vi "高速数据通信 指令批处理.vi"() -> ()   [LabVIEW 2018]
doc: "This example mainly indicates how to acquire profiles from controllers by using <B>Read Profiles (for High-Speed Communication)</B> VI via high-speed communication."
uses:
  Public/Clusters/Ethernet Config.ctl
  Public/Clusters/High-Speed Comm Start Req.ctl
  Public/Constants/High-Speed Comm Start Pos.ctl
  Public/Constants/High-Speed Receive Ratio.ctl
  Public/Clusters/Profile Info.ctl
  KEYENCE LJ-X8000A.lvlib
panel:
  in  "Program No":u8
  in  "btnChangeProgram":bool
  in  "stop measure":bool
  in  "start measure":bool
  out "Luminance Image":u16[][](graph)
  out "error out":errorcluster
  out "Comm":bool
  out "Monitoring":bool
  out "Timeout Cnt":u32
  out "Height Image":dbl[][](graph)
  out "Read Cnt":u32
  out "Notify":u32
  out "Buf Usage Rate":u32
  out "Profile Info":T1
  in  "Start Req":T2={"High-Speed Comm Start Pos"=2, "Read Profile Cnt"=11, "High-Speed Receive Ratio"=16} {"High-Speed Receive Ratio" items=["LOWEST"=0, "LOW"=16, "MIDDLE"=17, "HIGH"=18, "HIGHEST"=32]; "High-Speed Comm Start Pos" items=["SEND COMPLETE POS", "OLDEST", "NEXT"]}
  in  "Port No":u16=24692
  in  "Stop Monitoring":bool
  in  "Start Monitoring":bool
  in  "Stop High Speed Comm":bool
  in  "Start High Speed Comm":bool
  in  "Stop VI":bool
  in  "Ethernet Config":T5={"IP Address"=[192, 168, 0, 1], "Port No"=24691}
  # "High Speed Data Communication Start/Stop"
  # "Read Profiles Start/Stop"
  # "Communication Configuration"
  # "Output from Read Profiles VI"
  # "Communication Configuration\nfor High Speed Communication"
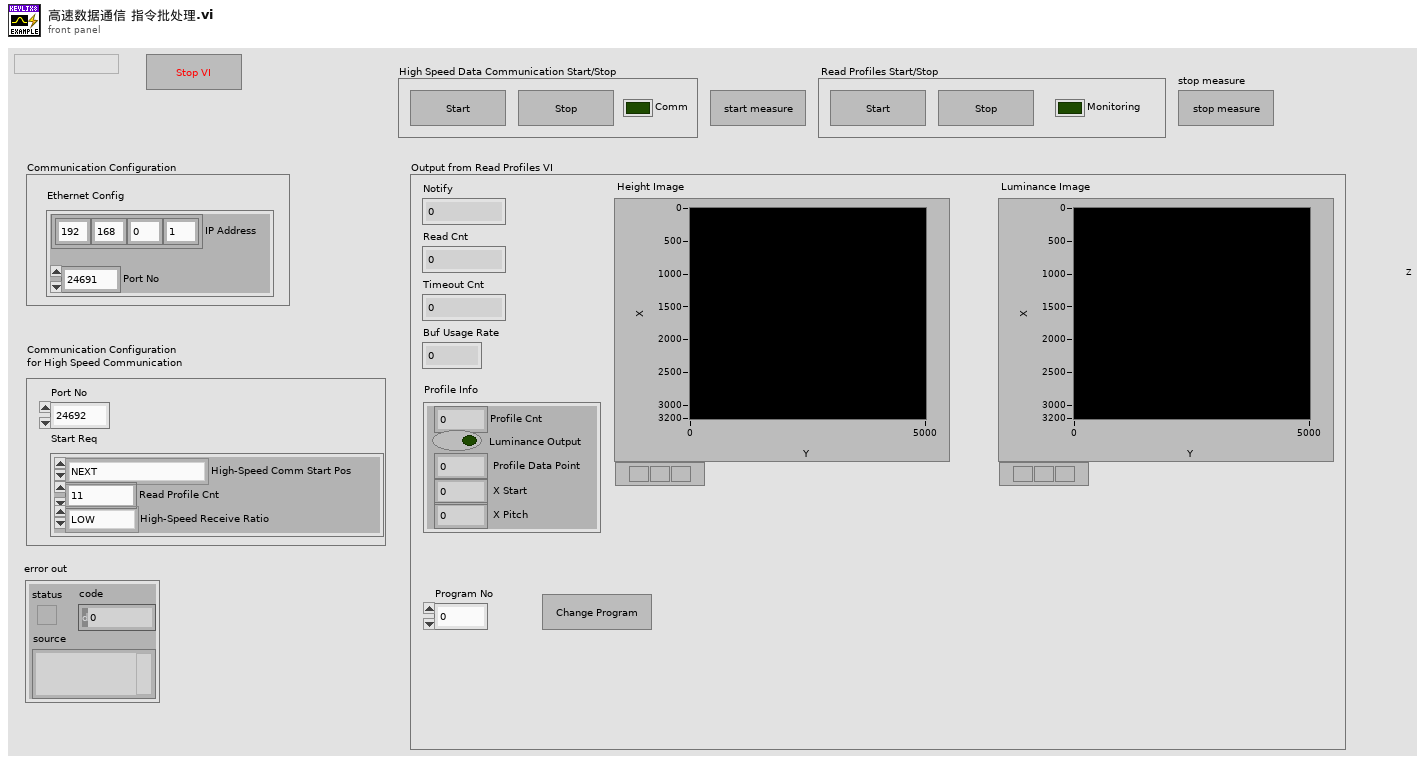
[diagram p1: front panel]
types:
  T1 = typedef "KEYENCE LJ-X8000A.lvlib/Profile Info.ctl" = cluster{"Profile Cnt":u8, "Luminance Output":bool, " Profile Data Point":u16, " X Start":i32, " X Pitch":i32}
  T2 = typedef "KEYENCE LJ-X8000A.lvlib/High-Speed Comm Start Req.ctl" = cluster{"High-Speed Comm Start Pos":T3, "Read Profile Cnt":u32, "High-Speed Receive Ratio":T4}
  T3 = typedef "KEYENCE LJ-X8000A.lvlib/High-Speed Comm Start Pos.ctl" = u8
  T4 = typedef "KEYENCE LJ-X8000A.lvlib/High-Speed Receive Ratio.ctl" = u8
  T5 = typedef "KEYENCE LJ-X8000A.lvlib/Ethernet Config.ctl" = cluster{"IP Address":u8[], "Port No":u16}
  T6 = enum8{"Enabled", "Disabled", "Disabled and Grayed Out"}
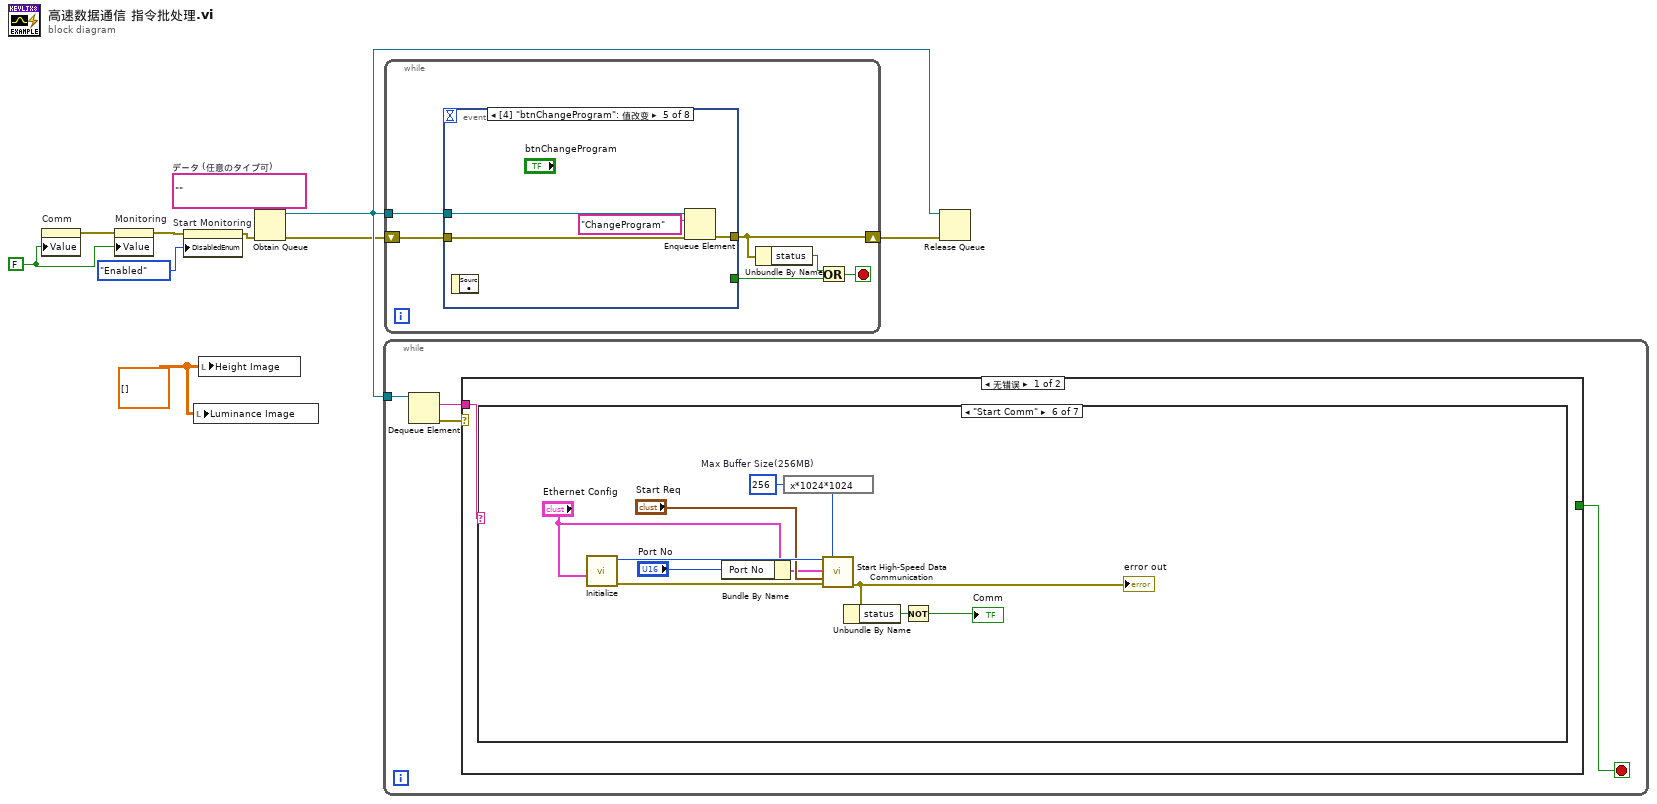
[diagram p0: block diagram]
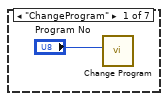
[diagram p2: hidden frame]
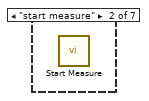
[diagram p3: hidden frame]
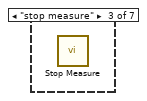
[diagram p4: hidden frame]
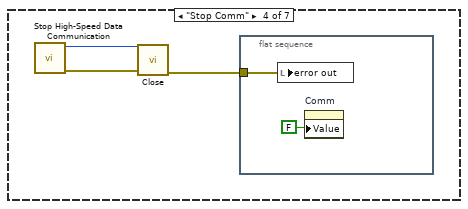
[diagram p5: hidden frame]
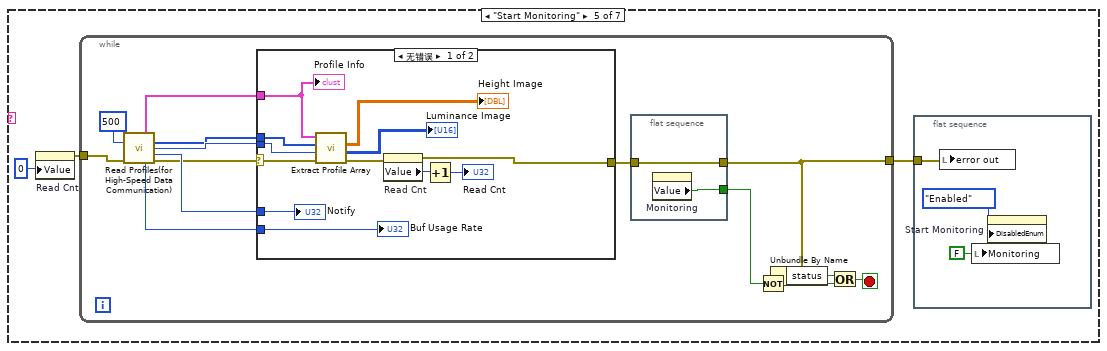
[diagram p6: hidden frame]
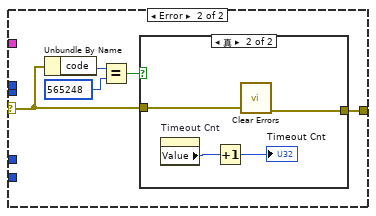
[diagram p7: hidden frame]
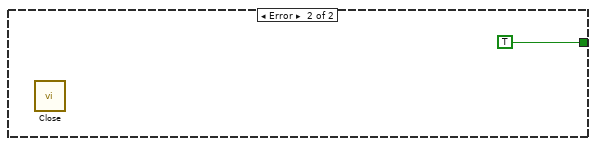
[diagram p10: hidden frame]
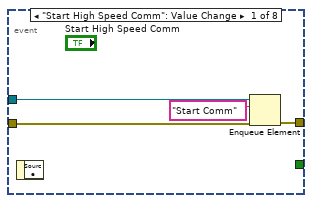
[diagram p11: hidden frame]
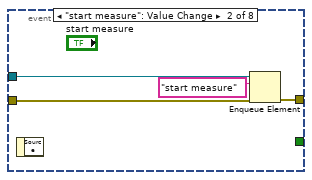
[diagram p12: hidden frame]
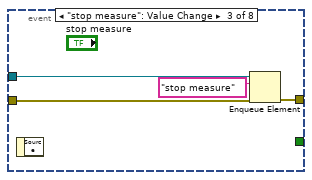
[diagram p13: hidden frame]
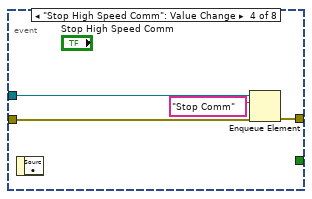
[diagram p14: hidden frame]
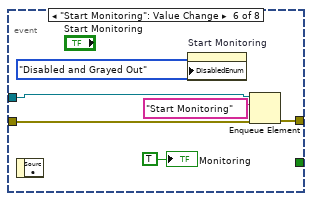
[diagram p15: hidden frame]
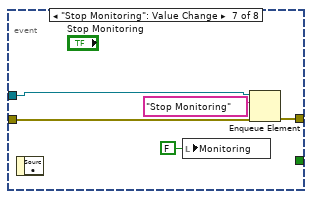
[diagram p16: hidden frame]
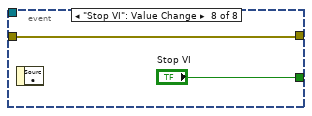
[diagram p17: hidden frame]
diagram:
  w1 = dbl[][] []
  w6 = FALSE ("Monitoring")
  w8 = ""  # データ (任意のタイプ可)
  n1 = property on="Comm" class="Bool (严格)"("Value"=w6) -> (error out=w7:errorcluster)  [unwired: 2 in, 1 out]
  n2 = property on="Monitoring" class="Bool (严格)"(error in=w7, "Value"=w6) -> (error out=w5:errorcluster)  [unwired: 1 in, 1 out]
  n3 = property on="Start Monitoring" class="Bool"(error in=w5, "DisabledEnum"=T6."Enabled" ("–³Œø")) -> (error out=w3:errorcluster)  [unwired: 1 in, 1 out]
  n4 = local write "Luminance Image"(w1) -> ()
  n5 = local write "Height Image"(w1) -> ()
  n6 = Obtain Queue(element data type=w8, error in (no error)=w3) -> (queue out=w9:refnum<queue>, error out=w4:errorcluster)  [unwired: 3 in, 1 out]
  n7 = while {
    tunnel: w9 -> [w14]
    stop <- w11 stop-if-true
    n8 = Dequeue Element(queue=w14) -> (element=w12:string, error out=w13:errorcluster)  [unwired: 2 in, 2 out]
    n9 = case shown="无错误" w13 {
      tunnel: w12 -> [w15 _]
      tunnel: [_ TRUE] -> w11
      frame No Error {
        n10 = case shown="\"Start Comm\"" w15 {
          frame "ChangeProgram" {
            n11 = call "Change Program.vi"("Program No"="Program No") -> ()  [unwired: 9 in, 2 out]
          }
          frame "start measure" {
            n12 = call "Start Measure.vi"() -> ()  [unwired: 10 in, 2 out]
          }
          frame "stop measure" {
            n13 = call "Stop Measure.vi"() -> ()  [unwired: 10 in, 2 out]
          }
          frame "Stop Comm" {
            n14 = call "Stop High-Speed Data Communication.vi"() -> ("error out"=w19:errorcluster, "Device ID out"=w18:i32)  [unwired: 10 in]
            n15 = call "Close.vi"("error in (no error)"=w19, "Device ID (0)"=w18) -> ("error out"=w17:errorcluster)  [unwired: 8 in, 1 out]
            n16 = flat-sequence {
              tunnel: w17 -> [w21]
              frame #0 {
                n17 = local write "error out"(w21) -> ()
                n18 = property on="Comm" class="Bool (严格)"("Value"=FALSE ("Comm")) -> ()  [unwired: 2 in, 2 out]
              }
            }
          }
          frame "Start Monitoring" {
            n19 = property on="Read Cnt" class="DigNum (严格)"("Value"=u32 0 ("Read Cnt")) -> (error out=w23:errorcluster)  [unwired: 2 in, 1 out]
            n20 = while {
              tunnel: w23 -> [w36]
              tunnel: [w31] -> w24
              stop <- w33 stop-if-true
              n21 = call "Read Profiles(for High-Speed Data Communication).vi"("Timeout"=u32 500, "error in (no error)"=w36) -> ("Profile Info"=w40:T1, "Profile Data"=w34:u32[], "Rsp Profile Cnt"=w37:u32, "Notify"=w38:u32, "Buf Usage Rate"=w41:u32, "error out"=w29:errorcluster)  [unwired: 7 in, 1 out]
              n22 = case shown="无错误" w29 {
                selector: w29 -> [w50 w60]
                tunnel: w41 -> [w55 _]
                tunnel: w40 -> [w49 _]
                tunnel: w38 -> [w54 _]
                tunnel: w37 -> [w47 _]
                tunnel: [w51 w59] -> w32
                tunnel: w34 -> [w48 _]
                frame No Error {
                  n23 = call "Extract Profile Array.vi"("error in (no error)"=w50, "Profile Cnt"=w47, "Profile Data"=w48, "Profile Info"=w49) -> ("error out"=w46:errorcluster, "Luminance Profile Array"=→"Luminance Image":u16[][], "Height Profile Array"=→"Height Image":dbl[][])  [unwired: 4 in, 1 out]
                  n24 = property on="Read Cnt" class="DigNum (严格)"(error in=w46) -> (error out=w51:errorcluster, "Value"=w53:u32)  [unwired: 1 in, 1 out]
                  n25 = Increment(x=w53) -> (x+1=→"Read Cnt":u32)
                  "Buf Usage Rate" <- w55
                  "Profile Info" <- w49
                  "Notify" <- w54
                }
                frame Error {
                  n26 = Unbundle By Name(w60) -> ("code"=w58:i32)
                  n27 = Equal?(x=w58, y=565248) -> (x = y?=w56:bool)
                  n28 = case shown="真" w56 {
                    tunnel: w60 -> [w61 w65]
                    tunnel: [w61 w64] -> w59
                    frame False {
                    }
                    frame True {
                      n29 = property on="Timeout Cnt" class="DigNum (严格)"() -> ("Value"=w63:u32)  [unwired: 2 in, 2 out]
                      n30 = Increment(x=w63) -> (x+1=→"Timeout Cnt":u32)
                      n31 = call <vilib>:"Clear Errors.vi"("error in (no error)"=w65) -> ("error out"=w64:errorcluster)  [unwired: 5 in, 1 out]
                    }
                  }
                }
              }
              n32 = flat-sequence {
                tunnel: w32 -> [w43]
                tunnel: [w43] -> w31
                tunnel: [w42] -> w30
                frame #0 {
                  n33 = property on="Monitoring" class="Bool (严格)"() -> ("Value"=w42:bool)  [unwired: 2 in, 2 out]
                }
              }
              n34 = Not(x=w30) -> (.not. x?=w35:bool)
              n35 = Unbundle By Name(w31) -> ("status"=w28:bool)
              n36 = Or(x=w28, y=w35) -> (x .or. y?=w33:bool)
            }
            n37 = flat-sequence {
              tunnel: w24 -> [w25]
              frame #0 {
                n38 = local write "error out"(w25) -> ()
                n39 = local write "Monitoring"(FALSE ("Monitoring")) -> ()
                n40 = property on="Start Monitoring" class="Bool"("DisabledEnum"=T6."Enabled" ("–³Œø")) -> ()  [unwired: 2 in, 2 out]
              }
            }
          }
          frame "Start Comm" {
            w67 = u32 256  # Max Buffer Size(256MB)
            n41 = call "Initialize.vi"("Ethernet Config"="Ethernet Config") -> ("error out"=w69:errorcluster, "Device ID out"=w76:i32)  [unwired: 9 in]
            n42 = Bundle By Name(cluster="Ethernet Config", "Port No"="Port No") -> (w72:T5)
            n43 = expression code="x*1024*1024"(w67) -> (w71:u32)
            n44 = call "Start High-Speed Data Communication.vi"("Device ID"=w76, "Max Buffer Size"=w71, "Ethernet Config"=w72, "Start Req"="Start Req", "error in (no error)"=w69) -> ("error out"=w68:errorcluster)  [unwired: 9 in, 1 out]
            "error out" <- w68
            n45 = Unbundle By Name(w68) -> ("status"=w66:bool)
            n46 = Not(x=w66) -> (.not. x?=→"Comm":bool)
          }
          frame Default {
          }
        }
      }
      frame Error {
        n47 = call "Close.vi"() -> ()  [unwired: 10 in, 2 out]
      }
    }
  }
  n48 = while {
    shift-right: [w79] -> w10
    shift-left: w4 -> [w82]
    tunnel: w9 -> [w83]
    stop <- w80 stop-if-true
    n49 = event shown="[4] \"btnChangeProgram\": 值改变" {
      selector: _ -> [_ _ _ _ _ _ _ _]
      dyn-events: _ -> [_ _ _ _ _ _ _ _]
      timeout: _ -> [_ _ _ _ _ _ _ _]
      tunnel: w83 -> [w87 w91 w95 w99 w103 w105 w110 _]
      tunnel: w82 -> [w86 w90 w94 w98 w102 w109 w114 w116]
      tunnel: [w85 w89 w93 w97 w101 w108 w113 w116] -> w79
      tunnel: [_ _ _ _ _ _ _ "Stop VI"] -> w81
      event "Start High Speed Comm": Value Change {
        n50 = event-data() -> ()  [unwired: 1 in, 1 out]
        n51 = Enqueue Element(queue=w87, element="Start Comm", error in (no error)=w86) -> (error out=w85:errorcluster)  [unwired: 1 in, 2 out]
      }
      event "start measure": Value Change {
        n52 = event-data() -> ()  [unwired: 1 in, 1 out]
        n53 = Enqueue Element(queue=w91, element="start measure", error in (no error)=w90) -> (error out=w89:errorcluster)  [unwired: 1 in, 2 out]
      }
      event "stop measure": Value Change {
        n54 = event-data() -> ()  [unwired: 1 in, 1 out]
        n55 = Enqueue Element(queue=w95, element="stop measure", error in (no error)=w94) -> (error out=w93:errorcluster)  [unwired: 1 in, 2 out]
      }
      event "Stop High Speed Comm": Value Change {
        n56 = event-data() -> ()  [unwired: 1 in, 1 out]
        n57 = Enqueue Element(queue=w99, element="Stop Comm", error in (no error)=w98) -> (error out=w97:errorcluster)  [unwired: 1 in, 2 out]
      }
      event "btnChangeProgram": Value Change {
        n58 = event-data() -> ()  [unwired: 1 in, 1 out]
        n59 = Enqueue Element(queue=w103, element="ChangeProgram", error in (no error)=w102) -> (error out=w101:errorcluster)  [unwired: 1 in, 2 out]
      }
      event "Start Monitoring": Value Change {
        n60 = event-data() -> ()  [unwired: 1 in, 1 out]
        n61 = property on="Start Monitoring" class="Bool"("DisabledEnum"=T6."Disabled and Grayed Out" ("–³Œø")) -> ()  [unwired: 2 in, 2 out]
        n62 = Enqueue Element(queue=w105, element="Start Monitoring", error in (no error)=w109) -> (error out=w108:errorcluster)  [unwired: 1 in, 2 out]
        "Monitoring" <- TRUE ("Monitoring")
      }
      event "Stop Monitoring": Value Change {
        n63 = event-data() -> ()  [unwired: 1 in, 1 out]
        n64 = local write "Monitoring"(FALSE ("Monitoring")) -> ()
        n65 = Enqueue Element(queue=w110, element="Stop Monitoring", error in (no error)=w114) -> (error out=w113:errorcluster)  [unwired: 1 in, 2 out]
      }
      event "Stop VI": Value Change {
        n66 = event-data() -> ()  [unwired: 1 in, 1 out]
      }
    }
    n67 = Unbundle By Name(w79) -> ("status"=w78:bool)
    n68 = Or(x=w78, y=w81) -> (x .or. y?=w80:bool)
  }
  n69 = Release Queue(queue=w9, error in (no error)=w10) -> ()  [unwired: 1 in, 3 out]
